vi "filters.vi"(6 "Counter Data":u32[][](array[numeric]), 8 "error in":errorcluster, 9 "lasers okay?":bool, 10 "Array of ROI sums":dbl[][](array[numeric]), 11 "Filter Cluster":T1) -> (0 "error out":errorcluster, 3 "All shots passed filters?":bool)   [LabVIEW 2013]
uses:
  filters.ctl
panel:
  out "counter data size(s)":i32[](array[numeric])
  # "Regions of Interest -->"
  # "Shots\n   |\n  V"
  # "Counters -->"
  # "Counter\n    bins\n       |\n      V"
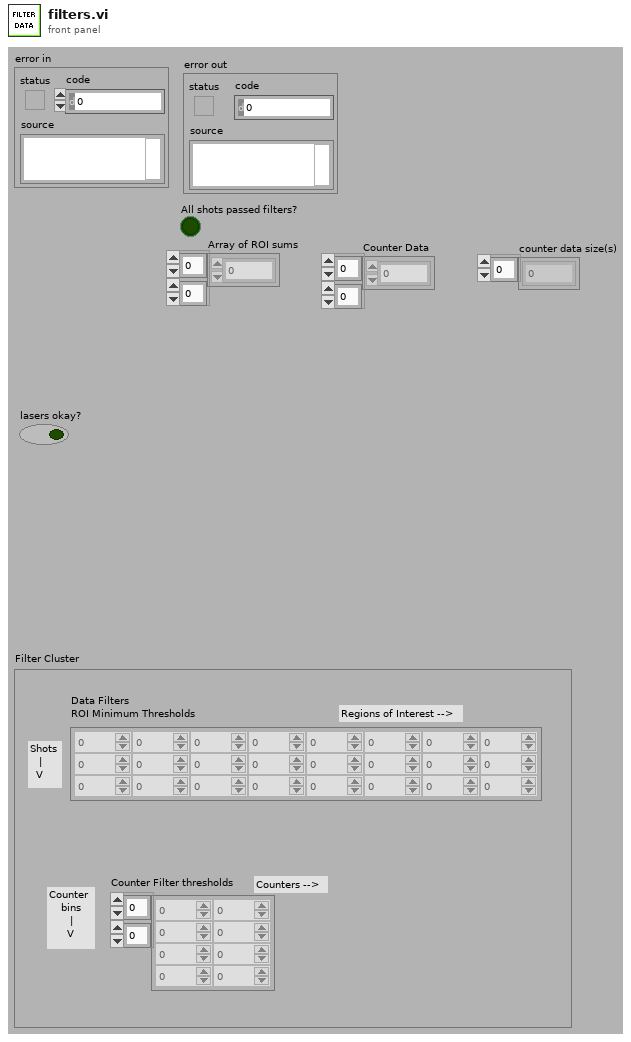
[diagram p1: front panel]
types:
  T1 = typedef "filters.ctl" = cluster{"Counter Filter thresholds":u32[][], "Data Filters\nROI Minimum Thresholds":u64[][]}
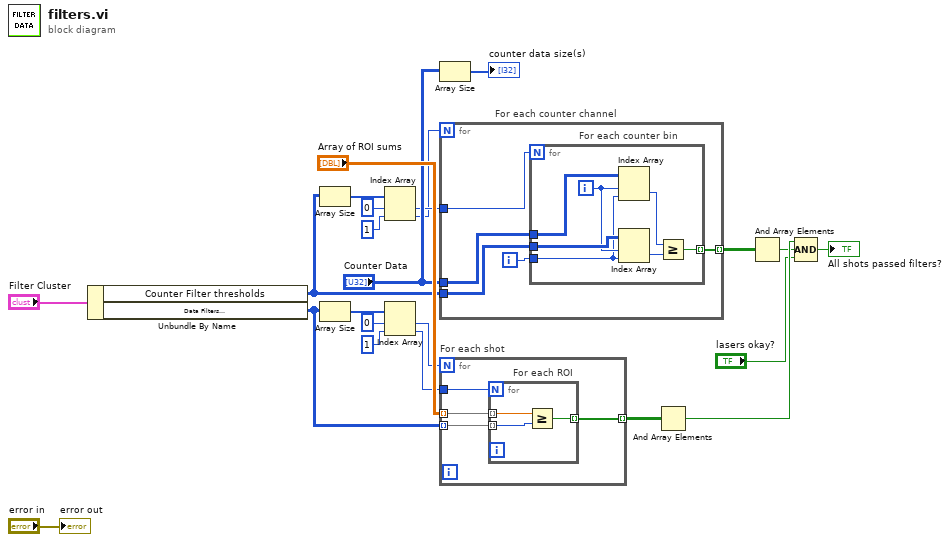
[diagram p0: block diagram]
diagram:
  n1 = Unbundle By Name("Filter Cluster") -> ("Counter Filter thresholds"=w6:u32[][], "Data Filters\nROI Minimum Thresholds"=w5:u64[][])
  n2 = Array Size(array=w6) -> (size(s)=w15:i32[])
  n3 = Array Size(array=w5) -> (size(s)=w21:i32[])
  n4 = Index Array(array=w15, index #1=0 ("index"), index #2=1 ("index")) -> (element #1=w9:i32, element #2=w8:i32)
  n5 = Index Array(array=w21, index #1=0 ("index"), index #2=1 ("index")) -> (element #1=w18:i32, element #2=w17:i32)
  n6 = Array Size(array="Counter Data") -> (size(s)=→"counter data size(s)":i32[])
  n7 = for "For each counter channel" {
    N: w8 -> [_]
    tunnel: [w28] -> w16 mode=indexing
    tunnel: "Counter Data" -> [w25]
    tunnel: w6 -> [w27]
    tunnel: w9 -> [w26]
    i -> [w24]
    n8 = for "For each counter bin" {
      N: w26 -> [_]
      tunnel: w27 -> [w32]
      tunnel: [w35] -> w28 mode=indexing
      tunnel: w25 -> [w34]
      tunnel: w24 -> [w29]
      i -> [w30]
      n9 = Index Array(array=w34, index (row)=w30, index (col)=w29) -> (element=w33:u32)
      n10 = Index Array(array=w32, index (row)=w30, index (col)=w29) -> (element=w31:u32)
      n11 = Greater Or Equal?(x=w33, y=w31) -> (x >= y?=w35:bool)
    }
  }
  n12 = for "For each shot" {
    N: w18 -> [_]
    tunnel: [w39] -> w23 mode=indexing
    tunnel: "Array of ROI sums" -> [w38] mode=indexing
    tunnel: w5 -> [w37] mode=indexing
    tunnel: w17 -> [w36]
    n13 = for "For each ROI" {
      N: w36 -> [_]
      tunnel: w38 -> [w41] mode=indexing
      tunnel: w37 -> [w42] mode=indexing
      tunnel: [w40] -> w39 mode=indexing
      n14 = Greater Or Equal?(x=w41, y=w42) -> (x >= y?=w40:bool)
    }
  }
  n15 = And Array Elements(Boolean array=w23) -> (logical AND=w4:bool)
  n16 = And Array Elements(Boolean array=w16) -> (logical AND=w3:bool)
  n17 = Compound Arithmetic op=AND(w4, w3, "lasers okay?") -> (→"All shots passed filters?":bool)
  "error out" <- "error in"
